vi "Turn Silver.vi"(8 "error in (no error)":errorcluster) -> (0 "error out":errorcluster)   [LabVIEW 2021]
uses:
  <vilib>/Utility/miscctls.llb/LVFontTypeDef.ctl
  <vilib>/Utility/miscctls.llb/LVPositionTypeDef.ctl
panel:
  out "Control Types on VI":string[](array[string])
  in  "vi path":path
  # "This VI will attempt to replace the front panel controls with their silver versions.  Not all controls are supported but you can follow the same steps to add support for other controls.\nNote that all DAQmx controls will be changed to Channel terminals, rather than Device terminals.\n\nThis VI is shamelessly stolen and edited from Hooovahh's great post here:\nhttps://forums.ni.com/t5/LabVIEW/Replace-cluster-bug/m-p/3148093/highlight/true#M906580"
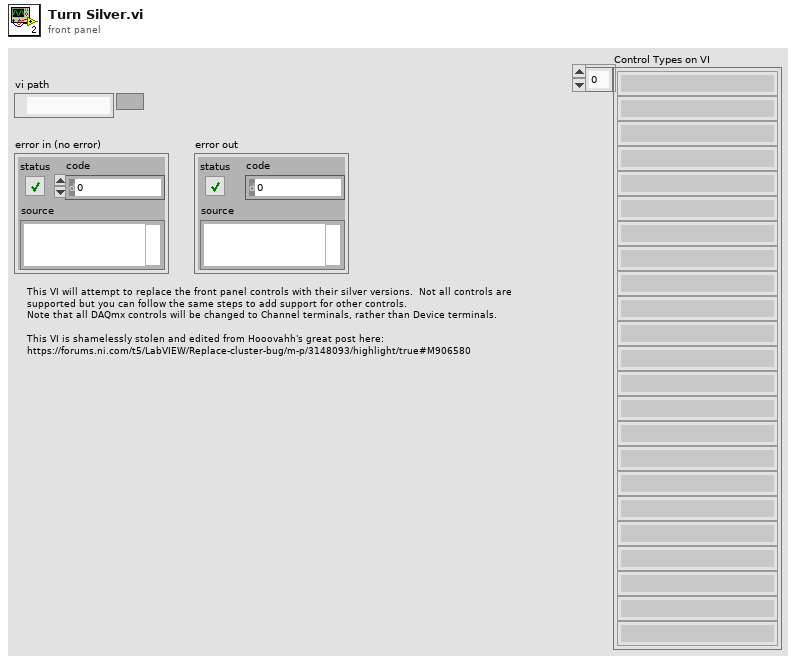
[diagram p1: front panel]
types:
  T1 = enum32{"Invalid", "Standard", "Closed", "Hidden", "Minimized", "Maximized"}
  T2 = typedef "LVFontTypeDef.ctl" = cluster{"Font Name":string, "Size":u16, "Bold":bool, "Italic":bool, "Underline":bool, "Strikeout":bool, "Color":u32}
  T3 = typedef "LVPositionTypeDef.ctl" = cluster{"Left":i32, "Top":i32}
  T4 = enum32{"not a typedef", "typedef", "strict typedef", "class private data"}
  T5 = typedef "LVBrowseOptionsTypeDef.ctl" = cluster{"Prompt":string, "Match Pattern":string, "select mode":enum32{"existing file", "new file", "new or existing file", "existing dir", "new dir", "new or existing dir", "existing file (use LLBs)", "new file (use LLBs)", "new or existing file (use LLBs)", "new or existing file or directory (use LLBs)", "existing dir (use LLBs)", "new dir (use LLBs)", "new or existing dir (use LLBs)", "existing file or dir", "new file or dir", "new or existing file or dir", "existing file or dir (use LLBs)", "new file or dir (use LLBs)"}, "Start Path":path, "Pattern Label":string, "Button Text":string}
  T6 = cluster{"left":i16, "top":i16, "right":i16, "bottom":i16}
  T7 = typedef "LVStringsAndValuesArrayTypeDef.ctl" = cluster{"String":string, "Value":ext}[]
  T8 = typedef "LVBoundsTypeDef.ctl" = cluster{"Width":u32, "Height":u32}
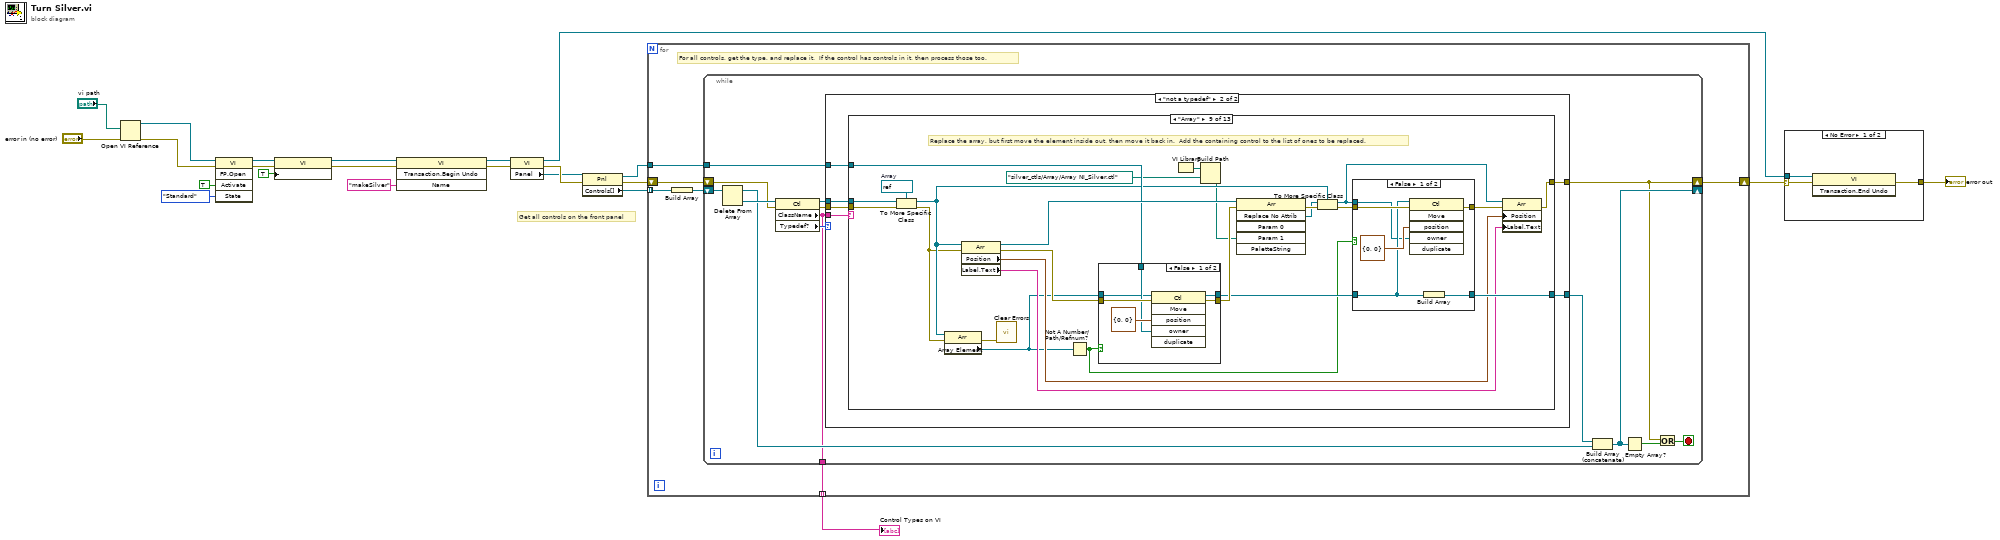
[diagram p0: block diagram]
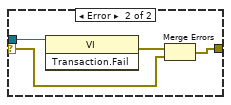
[diagram p2: hidden frame]
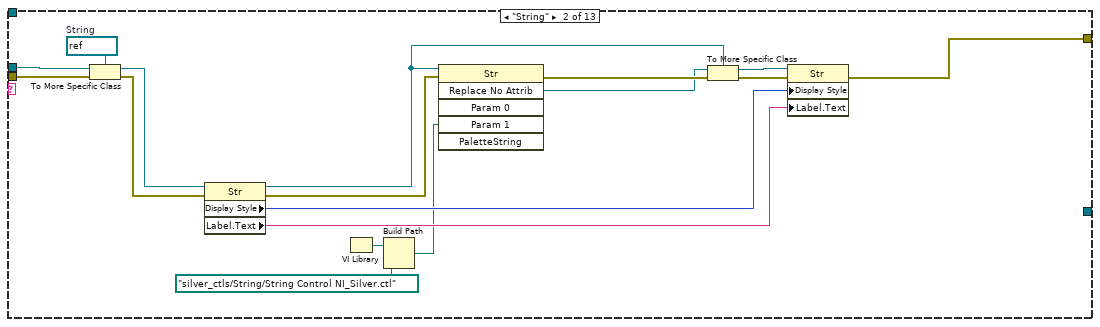
[diagram p5: hidden frame]
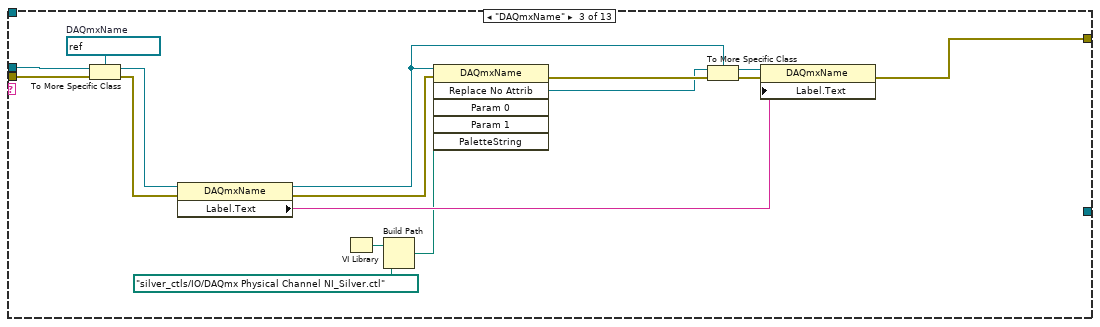
[diagram p6: hidden frame]
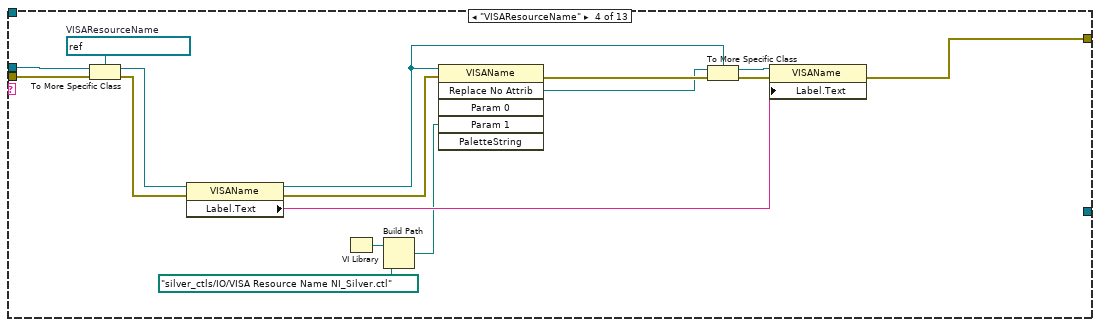
[diagram p7: hidden frame]
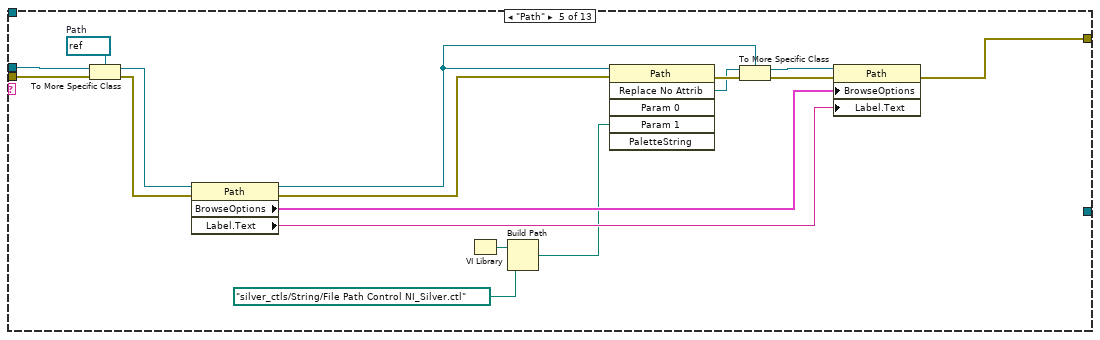
[diagram p8: hidden frame]
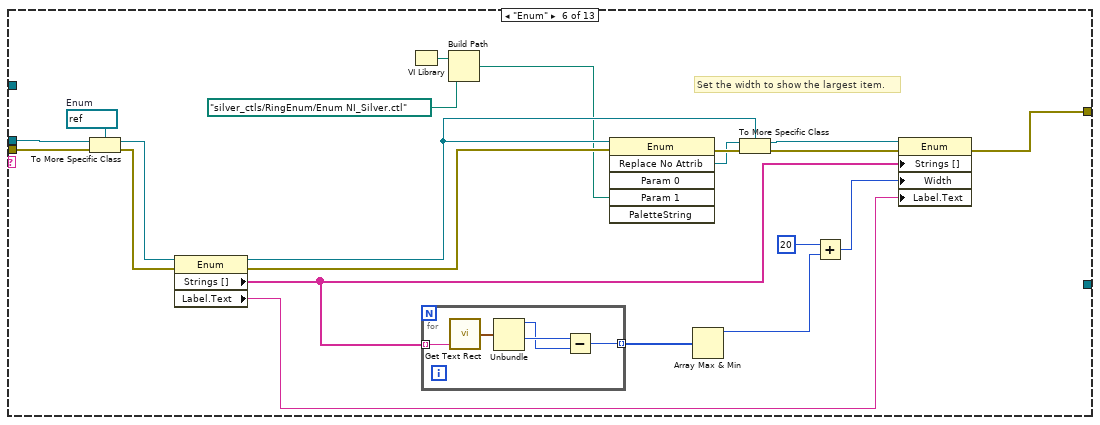
[diagram p9: hidden frame]
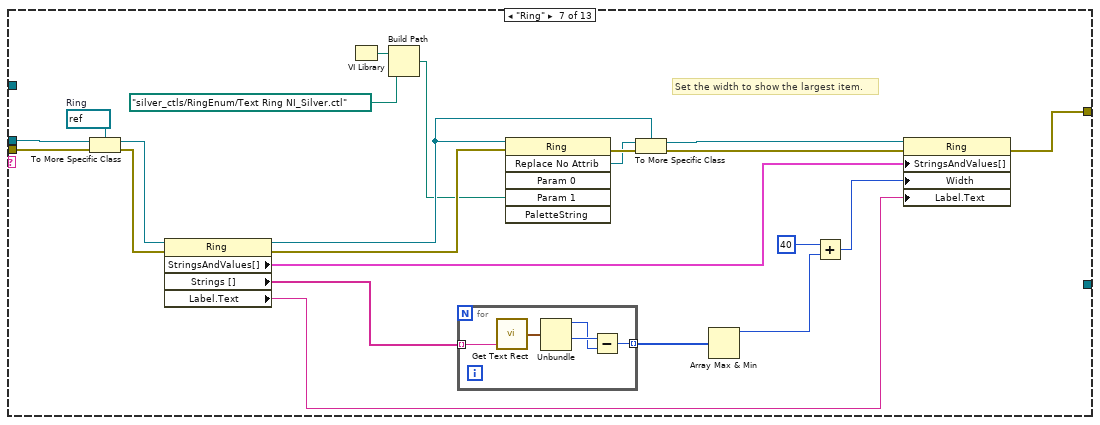
[diagram p10: hidden frame]
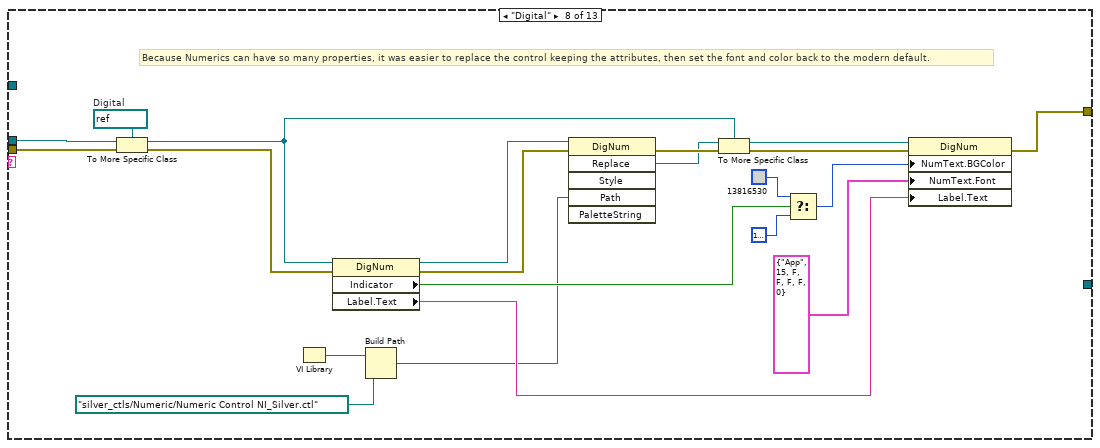
[diagram p11: hidden frame]
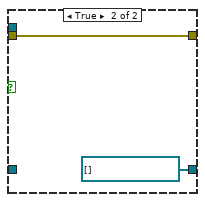
[diagram p12: hidden frame]
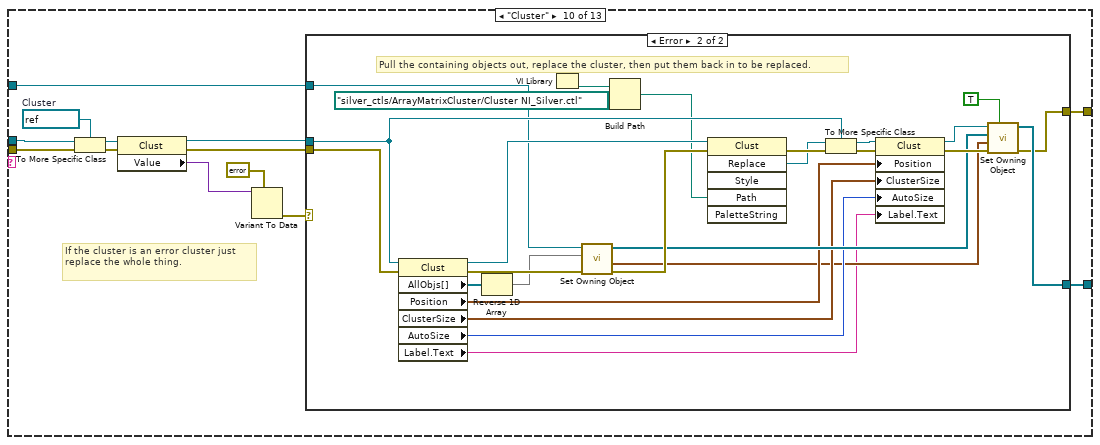
[diagram p14: hidden frame]
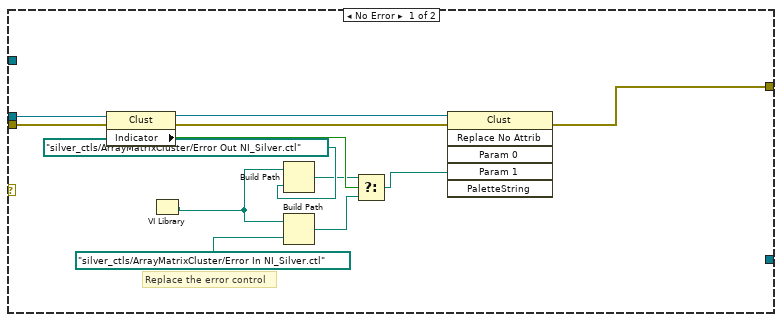
[diagram p15: hidden frame]
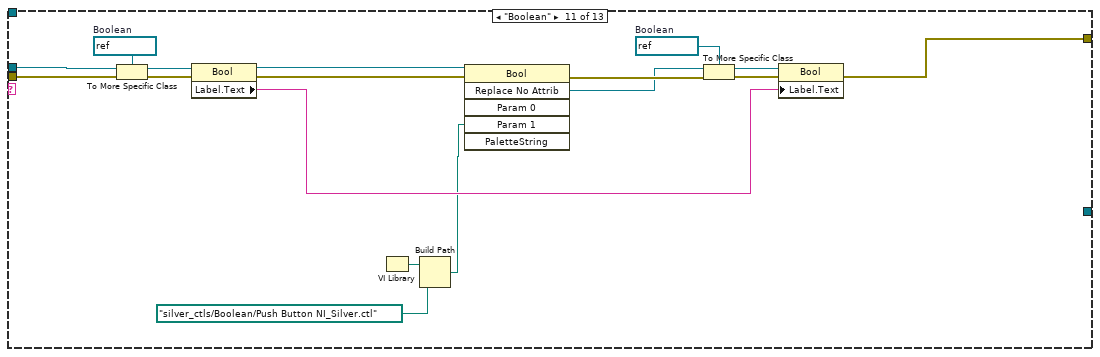
[diagram p16: hidden frame]
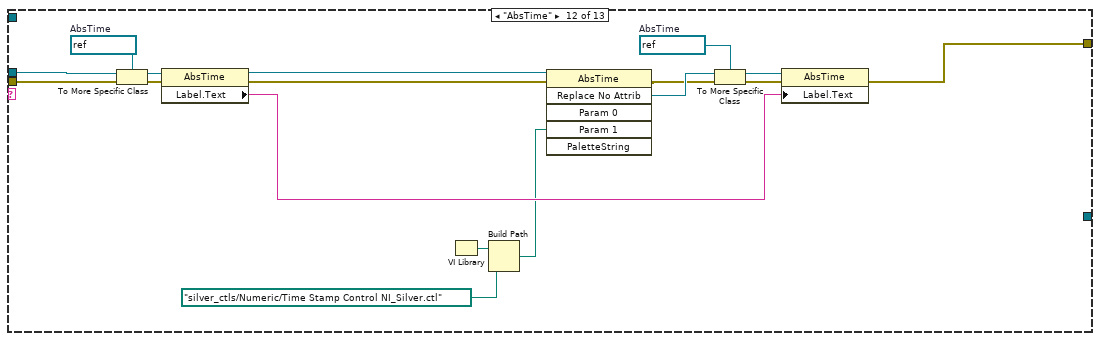
[diagram p17: hidden frame]
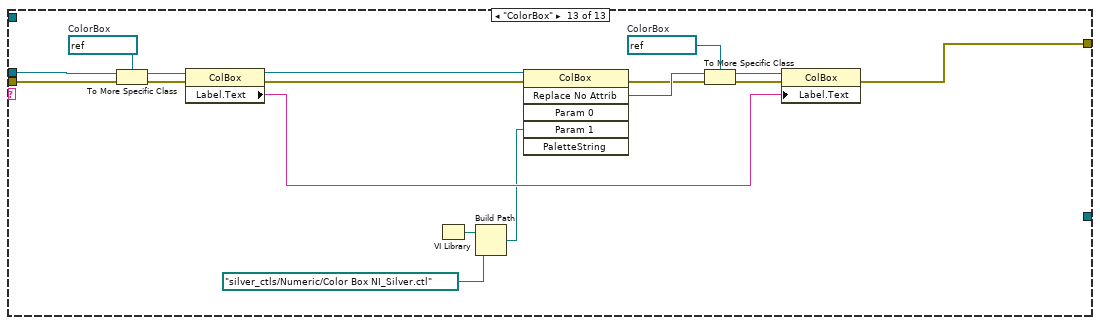
[diagram p18: hidden frame]
diagram:
  # "Get all controls on the front panel"
  n1 = Open VI Reference(vi path="vi path", error in (no error)="error in (no error)") -> (vi reference=w5:refnum<vi>, error out=w3:errorcluster)  [unwired: 4 in]
  n2 = invoke class="VI" method="FP.Open"(reference=w5, error in=w3, "Activate"=TRUE ("Activate?"), "State"=T1."Standard") -> (reference out=w11:refnum<vi>, error out=w12:errorcluster)  [unwired: 1 in, 3 out]
  n3 = property class="VI"(reference=w11, error in=w12, "Front Panel.IsFrontmost"=TRUE ("Front Panel Window:Is Frontmost")) -> (reference out=w6:refnum<vi>, error out=w7:errorcluster)
  n4 = invoke class="VI" method="Transaction.Begin Undo"(reference=w6, error in=w7, "Name"="makeSilver") -> (reference out=w17:refnum<vi>, error out=w18:errorcluster)  [unwired: 1 in, 2 out]
  n5 = property class="VI"(reference=w17, error in=w18) -> (reference out=w14:refnum<vi>, error out=w21:errorcluster, "Panel"=w20:refnum<vi>)
  n6 = property class="Pnl"(reference=w20, error in=w21) -> (reference out=w19:refnum<vi>, error out=w22:errorcluster, "Controls[]"=w23:refnum<vi>[])
  n7 = for {
    tunnel: w23 -> [w28] mode=indexing
    tunnel: w19 -> [w29]
    shift-right: [w25] -> w13
    shift-left: w22 -> [w26]
    tunnel: [w24] -> w1 mode=indexing
    # "For all controls, get the type, and replace it.  If the control has controls in it, then process those too."
    n8 = Build Array(w28) -> (w27:refnum<vi>[])
    n9 = while {
      tunnel: w29 -> [w43]
      shift-right: [w34] -> _
      shift-left: w27 -> [w38]
      shift-right: [w31] -> w25
      shift-left: w26 -> [w33]
      tunnel: [w30] -> w24
      stop <- w32 stop-if-true
      n10 = Delete From Array(array=w38) -> (deleted portion=w37:refnum<vi>, array with subset deleted=w35:refnum<vi>[])  [unwired: 2 in]
      n11 = property class="Ctl"(reference=w37, error in=w33) -> (reference out=w42:refnum<vi>, error out=w41:errorcluster, "ClassName"=w30:string, "Typedef?"=w40:T4)
      n12 = case shown="\"not a typedef\"" w40 {
        tunnel: w43 -> [_ w50]
        tunnel: w42 -> [_ w49]
        tunnel: w30 -> [_ w48]
        tunnel: w41 -> [w44 w47]
        tunnel: [_ w46] -> w36
        tunnel: [w44 w45] -> w31
        frame Default {
          # "Don't try to replace type defs."
        }
        frame "not a typedef" {
          n13 = case shown="\"Array\"" w48 {
            tunnel: w50 -> [_ _ _ _ _ _ _ _ w207 w241 _ _ _]
            tunnel: w49 -> [_ w68 w84 w100 w117 w138 w165 w191 w216 w245 w300 w317 w334]
            tunnel: w47 -> [w51 w62 w78 w94 w111 w134 w161 w187 w212 w243 w297 w314 w331]
            tunnel: [_ _ _ _ _ _ _ _ w205 w240 _ _ _] -> w46
            tunnel: [w51 w55 w72 w88 w104 w121 w147 w175 w201 w233 w288 w304 w321] -> w45
            frame Default {
            }
            frame "String" {
              w67 = refnum<vi> refnum  # String
              n14 = To More Specific Class(target class=w67, reference=w68, error in=w62) -> (specific class reference=w58:refnum<vi>, error out=w60:errorcluster)
              n15 = property class="Str"(reference=w58, error in=w60) -> (reference out=w57:refnum<vi>, error out=w59:errorcluster, "Display Style"=w61:u32, "Label.Text"=w56:string)
              n16 = VI Library() -> (path=w53:path)
              n17 = Build Path(base path=w53, name or relative path=path "silver_ctls/String/String Control NI_Silver.ctl" ("path")) -> (appended path=w52:path)
              n18 = invoke class="Str" method="Replace No Attrib"(reference=w57, error in=w59, "Param 1"=w52) -> (error out=w66:errorcluster, "RepNoAttrib"=w64:refnum<vi>)  [unwired: 3 in, 4 out]
              n19 = To More Specific Class(target class=w57, reference=w64, error in=w66) -> (specific class reference=w63:refnum<vi>, error out=w65:errorcluster)
              n20 = property class="Str"(reference=w63, error in=w65, "Display Style"=w61, "Label.Text"=w56) -> (error out=w55:errorcluster)  [unwired: 1 out]
            }
            frame "DAQmxName" {
              w83 = refnum<vi> refnum  # DAQmxName
              n21 = To More Specific Class(target class=w83, reference=w84, error in=w78) -> (specific class reference=w75:refnum<vi>, error out=w77:errorcluster)
              n22 = property class="DAQmxName"(reference=w75, error in=w77) -> (reference out=w74:refnum<vi>, error out=w76:errorcluster, "Label.Text"=w73:string)
              n23 = VI Library() -> (path=w70:path)
              n24 = Build Path(base path=w70, name or relative path=path "silver_ctls/IO/DAQmx Physical Channel NI_Silver.ctl" ("path")) -> (appended path=w69:path)
              n25 = invoke class="DAQmxName" method="Replace No Attrib"(reference=w74, error in=w76, "Param 1"=w69) -> (error out=w82:errorcluster, "RepNoAttrib"=w80:refnum<vi>)  [unwired: 3 in, 4 out]
              n26 = To More Specific Class(target class=w74, reference=w80, error in=w82) -> (specific class reference=w79:refnum<vi>, error out=w81:errorcluster)
              n27 = property class="DAQmxName"(reference=w79, error in=w81, "Label.Text"=w73) -> (error out=w72:errorcluster)  [unwired: 1 out]
            }
            frame "VISAResourceName" {
              w99 = refnum<vi> refnum  # VISAResourceName
              n28 = To More Specific Class(target class=w99, reference=w100, error in=w94) -> (specific class reference=w91:refnum<vi>, error out=w93:errorcluster)
              n29 = property class="VISAName"(reference=w91, error in=w93) -> (reference out=w90:refnum<vi>, error out=w92:errorcluster, "Label.Text"=w89:string)
              n30 = VI Library() -> (path=w86:path)
              n31 = Build Path(base path=w86, name or relative path=path "silver_ctls/IO/VISA Resource Name NI_Silver.ctl" ("path")) -> (appended path=w85:path)
              n32 = invoke class="VISAName" method="Replace No Attrib"(reference=w90, error in=w92, "Param 1"=w85) -> (error out=w98:errorcluster, "RepNoAttrib"=w96:refnum<vi>)  [unwired: 3 in, 4 out]
              n33 = To More Specific Class(target class=w90, reference=w96, error in=w98) -> (specific class reference=w95:refnum<vi>, error out=w97:errorcluster)
              n34 = property class="VISAName"(reference=w95, error in=w97, "Label.Text"=w89) -> (error out=w88:errorcluster)  [unwired: 1 out]
            }
            frame "Path" {
              w116 = refnum<vi> refnum  # Path
              n35 = To More Specific Class(target class=w116, reference=w117, error in=w111) -> (specific class reference=w107:refnum<vi>, error out=w109:errorcluster)
              n36 = property class="Path"(reference=w107, error in=w109) -> (reference out=w106:refnum<vi>, error out=w108:errorcluster, "BrowseOptions"=w110:T5, "Label.Text"=w105:string)
              n37 = VI Library() -> (path=w102:path)
              n38 = Build Path(base path=w102, name or relative path=path "silver_ctls/String/File Path Control NI_Silver.ctl" ("path")) -> (appended path=w101:path)
              n39 = invoke class="Path" method="Replace No Attrib"(reference=w106, error in=w108, "Param 1"=w101) -> (error out=w115:errorcluster, "RepNoAttrib"=w113:refnum<vi>)  [unwired: 3 in, 4 out]
              n40 = To More Specific Class(target class=w106, reference=w113, error in=w115) -> (specific class reference=w112:refnum<vi>, error out=w114:errorcluster)
              n41 = property class="Path"(reference=w112, error in=w114, "BrowseOptions"=w110, "Label.Text"=w105) -> (error out=w104:errorcluster)  [unwired: 1 out]
            }
            frame "Enum" {
              w137 = refnum<vi> refnum  # Enum
              # "Set the width to show the largest item."
              n42 = To More Specific Class(target class=w137, reference=w138, error in=w134) -> (specific class reference=w131:refnum<vi>, error out=w133:errorcluster)
              n43 = property class="Enum"(reference=w131, error in=w133) -> (reference out=w130:refnum<vi>, error out=w132:errorcluster, "Strings []"=w127:string[], "Label.Text"=w122:string)
              n44 = VI Library() -> (path=w119:path)
              n45 = for {
                tunnel: w127 -> [w143] mode=indexing
                tunnel: [w139] -> w126 mode=indexing
                n46 = call <vilib>:"Get Text Rect.vi"("text"=w143) -> ("rect"=w140:T6)  [unwired: 8 in]
                n47 = Unbundle(w140) -> ("left"=w141:i16, "right"=w142:i16)  [unwired: 2 out]
                n48 = Subtract(x=w142, y=w141) -> (x-y=w139:i16)
              }
              n49 = Build Path(base path=w119, name or relative path=path "silver_ctls/RingEnum/Enum NI_Silver.ctl" ("path")) -> (appended path=w118:path)
              n50 = invoke class="Enum" method="Replace No Attrib"(reference=w130, error in=w132, "Param 1"=w118) -> (error out=w136:errorcluster, "RepNoAttrib"=w135:refnum<vi>)  [unwired: 3 in, 4 out]
              n51 = Array Max & Min(array=w126) -> (max value=w125:i16)  [unwired: 3 out]
              n52 = To More Specific Class(target class=w130, reference=w135, error in=w136) -> (specific class reference=w129:refnum<vi>, error out=w128:errorcluster)
              n53 = Add(x=i16 20, y=w125) -> (x+y=w124:i16)
              n54 = property class="Enum"(reference=w129, error in=w128, "Strings []"=w127, "Width"=w124, "Label.Text"=w122) -> (error out=w121:errorcluster)  [unwired: 1 out]
            }
            frame "Ring" {
              w164 = refnum<vi> refnum  # Ring
              # "Set the width to show the largest item."
              n55 = To More Specific Class(target class=w164, reference=w165, error in=w161) -> (specific class reference=w158:refnum<vi>, error out=w160:errorcluster)
              n56 = property class="Ring"(reference=w158, error in=w160) -> (reference out=w157:refnum<vi>, error out=w159:errorcluster, "StringsAndValues[]"=w149:T7, "Strings []"=w150:string[], "Label.Text"=w148:string)
              n57 = VI Library() -> (path=w145:path)
              n58 = Build Path(base path=w145, name or relative path=path "silver_ctls/RingEnum/Text Ring NI_Silver.ctl" ("path")) -> (appended path=w144:path)
              n59 = for {
                tunnel: w150 -> [w170] mode=indexing
                tunnel: [w166] -> w154 mode=indexing
                n60 = call <vilib>:"Get Text Rect.vi"("text"=w170) -> ("rect"=w167:T6)  [unwired: 8 in]
                n61 = Unbundle(w167) -> ("left"=w168:i16, "right"=w169:i16)  [unwired: 2 out]
                n62 = Subtract(x=w169, y=w168) -> (x-y=w166:i16)
              }
              n63 = invoke class="Ring" method="Replace No Attrib"(reference=w157, error in=w159, "Param 1"=w144) -> (error out=w163:errorcluster, "RepNoAttrib"=w162:refnum<vi>)  [unwired: 3 in, 4 out]
              n64 = To More Specific Class(target class=w157, reference=w162, error in=w163) -> (specific class reference=w156:refnum<vi>, error out=w155:errorcluster)
              n65 = Array Max & Min(array=w154) -> (max value=w153:i16)  [unwired: 3 out]
              n66 = Add(x=i16 40, y=w153) -> (x+y=w152:i16)
              n67 = property class="Ring"(reference=w156, error in=w155, "StringsAndValues[]"=w149, "Width"=w152, "Label.Text"=w148) -> (error out=w147:errorcluster)  [unwired: 1 out]
            }
            frame "Digital" {
              w190 = refnum<vi> refnum  # Digital
              # "Because Numerics can have so many properties, it was easier to replace the control keeping the attributes, then set the font and color back to the modern default."
              n68 = To More Specific Class(target class=w190, reference=w191, error in=w187) -> (specific class reference=w179:refnum<vi>, error out=w177:errorcluster)
              n69 = VI Library() -> (path=w172:path)
              n70 = property class="DigNum"(reference=w179, error in=w177) -> (reference out=w178:refnum<vi>, error out=w176:errorcluster, "Indicator"=w183:bool, "Label.Text"=w174:string)
              n71 = Build Path(base path=w172, name or relative path=path "silver_ctls/Numeric/Numeric Control NI_Silver.ctl" ("path")) -> (appended path=w171:path)
              n72 = invoke class="DigNum" method="Replace"(reference=w178, error in=w176, "Path"=w171) -> (error out=w189:errorcluster, "Replace"=w188:refnum<vi>)  [unwired: 3 in, 4 out]
              n73 = To More Specific Class(target class=w179, reference=w188, error in=w189) -> (specific class reference=w185:refnum<vi>, error out=w186:errorcluster)
              n74 = Select(t=u32 13816530, s=w183, f=u32 16777226) -> (s? t:f=w180:u32)
              n75 = property class="DigNum"(reference=w185, error in=w186, "NumText.BGColor"=w180, "NumText.Font"=T2 {"Font Name"="App", "Size"=15, "Bold"=FALSE, "Italic"=FALSE, "Underline"=FALSE, "Strikeout"=FALSE, "Color"=0} ("Numeric Text.Font"), "Label.Text"=w174) -> (error out=w175:errorcluster)  [unwired: 1 out]
            }
            frame "Array" {
              w215 = refnum<vi> refnum  # Array
              # "Replace the array, but first move the element inside out, then move it back in.  Add the containing control to the list of ones to be replaced."
              n76 = To More Specific Class(target class=w215, reference=w216, error in=w212) -> (specific class reference=w200:refnum<vi>, error out=w199:errorcluster)
              n77 = property class="Arr"(reference=w200, error in=w199) -> (error out=w195:errorcluster, "Array Element"=w198:refnum<vi>)  [unwired: 1 out]
              n78 = property class="Arr"(reference=w200, error in=w199) -> (reference out=w211:refnum<vi>, error out=w210:errorcluster, "Position"=w203:T3, "Label.Text"=w202:string)
              n79 = call <vilib>:"Clear Errors.vi"("error in (no error)"=w195) -> ()  [unwired: 5 in, 2 out]
              n80 = Not A Number/Path/Refnum?(number/path/refnum=w198) -> (NaN/Path/Refnum?=w196:bool)
              n81 = case shown="False" w196 {
                tunnel: w210 -> [w230 w232]
                tunnel: [w229 w232] -> w209
                tunnel: w207 -> [w227 _]
                tunnel: [w226 w231] -> w206
                tunnel: w198 -> [w225 w231]
                frame False {
                  n82 = invoke class="Ctl" method="Move"(reference=w225, error in=w230, "position"=T3 {"Left"=0, "Top"=0}, "owner"=w227) -> (reference out=w226:refnum<vi>, error out=w229:errorcluster)  [unwired: 2 in, 4 out]
                }
                frame True {
                }
              }
              n83 = VI Library() -> (path=w193:path)
              n84 = Build Path(base path=w193, name or relative path=path "silver_ctls/Array/Array NI_Silver.ctl" ("path")) -> (appended path=w192:path)
              n85 = invoke class="Arr" method="Replace No Attrib"(reference=w211, error in=w209, "Param 1"=w192) -> (error out=w214:errorcluster, "RepNoAttrib"=w213:refnum<vi>)  [unwired: 3 in, 4 out]
              n86 = To More Specific Class(target class=w200, reference=w213, error in=w214) -> (specific class reference=w197:refnum<vi>, error out=w208:errorcluster)
              n87 = case shown="False" w196 {
                tunnel: w208 -> [w221 w224]
                tunnel: w206 -> [w220 _]
                tunnel: [w219 refnum<vi>[] []] -> w205
                tunnel: w197 -> [w218 _]
                tunnel: [w217 w224] -> w204
                frame False {
                  n88 = invoke class="Ctl" method="Move"(reference=w220, error in=w221, "position"=T3 {"Left"=0, "Top"=0}, "owner"=w218) -> (error out=w217:errorcluster)  [unwired: 2 in, 5 out]
                  n89 = Build Array(w220) -> (w219:refnum<vi>[])
                }
                frame True {
                }
              }
              n90 = property class="Arr"(reference=w197, error in=w204, "Position"=w203, "Label.Text"=w202) -> (error out=w201:errorcluster)  [unwired: 1 out]
            }
            frame "Cluster" {
              w244 = refnum<vi> refnum  # Cluster
              # "If the cluster is an error cluster just replace the whole thing."
              n91 = To More Specific Class(target class=w244, reference=w245, error in=w243) -> (specific class reference=w238:refnum<vi>, error out=w242:errorcluster)
              n92 = property class="Clust"(reference=w238, error in=w242) -> (reference out=w237:refnum<vi>, error out=w239:errorcluster, "Value"=w236:variant)
              n93 = Variant To Data(type=errorcluster {"status"=FALSE, "code"=0, "source"=""} ("error in (no error)"), Variant=w236) -> (error out=w234:errorcluster)  [unwired: 1 in, 1 out]
              n94 = case shown="Error" w234 {
                tunnel: w237 -> [w255 w281]
                tunnel: w239 -> [w257 w279]
                tunnel: w241 -> [_ w276]
                tunnel: [_ w264] -> w240
                tunnel: [w247 w262] -> w233
                frame No Error {
                  # "Replace the error control"
                  n95 = property class="Clust"(reference=w255, error in=w257) -> (reference out=w254:refnum<vi>, error out=w256:errorcluster, "Indicator"=w251:bool)
                  n96 = VI Library() -> (path=w246:path)
                  n97 = Build Path(base path=w246, name or relative path=path "silver_ctls/ArrayMatrixCluster/Error Out NI_Silver.ctl") -> (appended path=w250:path)
                  n98 = Build Path(base path=w246, name or relative path=path "silver_ctls/ArrayMatrixCluster/Error In NI_Silver.ctl") -> (appended path=w249:path)
                  n99 = Select(t=w250, s=w251, f=w249) -> (s? t:f=w248:path)
                  n100 = invoke class="Clust" method="Replace No Attrib"(reference=w254, error in=w256, "Param 1"=w248) -> (error out=w247:errorcluster)  [unwired: 3 in, 5 out]
                }
                frame Error {
                  # "Pull the containing objects out, replace the cluster, then put them back in to be replaced."
                  n101 = property class="Clust"(reference=w281, error in=w279) -> (reference out=w280:refnum<vi>, error out=w278:errorcluster, "AllObjs[]"=w266:refnum<vi>[], "Position"=w269:T3, "ClusterSize"=w270:T8, "AutoSize"=w271:u32, "Label.Text"=w261:string)
                  n102 = Reverse 1D Array(array=w266) -> (reversed array=w263:refnum<vi>[])
                  n103 = VI Library() -> (path=w259:path)
                  n104 = call "Set Owning Object.vi"("error in (no error)"=w278, "All Controls In"=w263, "Owner Object"=w276) -> ("error out"=w277:errorcluster, "Positions"=w268:T3[], "All Controls Out"=w272:refnum<vi>[])  [unwired: 6 in]
                  n105 = Build Path(base path=w259, name or relative path=path "silver_ctls/ArrayMatrixCluster/Cluster NI_Silver.ctl") -> (appended path=w258:path)
                  n106 = invoke class="Clust" method="Replace"(reference=w280, error in=w277, "Path"=w258) -> (error out=w283:errorcluster, "Replace"=w282:refnum<vi>)  [unwired: 3 in, 4 out]
                  n107 = To More Specific Class(target class=w281, reference=w282, error in=w283) -> (specific class reference=w275:refnum<vi>, error out=w274:errorcluster)
                  n108 = property class="Clust"(reference=w275, error in=w274, "Position"=w269, "ClusterSize"=w270, "AutoSize"=w271, "Label.Text"=w261) -> (reference out=w265:refnum<vi>, error out=w273:errorcluster)
                  n109 = call "Set Owning Object.vi"("Set Absolute"=TRUE, "error in (no error)"=w273, "Absolute Positions"=w268, "All Controls In"=w272, "Owner Object"=w265) -> ("error out"=w262:errorcluster, "All Controls Out"=w264:refnum<vi>[])  [unwired: 4 in, 1 out]
                }
              }
            }
            frame "Boolean" {
              w291 = refnum<vi> refnum  # Boolean
              w299 = refnum<vi> refnum  # Boolean
              n110 = To More Specific Class(target class=w299, reference=w300, error in=w297) -> (specific class reference=w295:refnum<vi>, error out=w298:errorcluster)
              n111 = property class="Bool"(reference=w295, error in=w298) -> (reference out=w294:refnum<vi>, error out=w296:errorcluster, "Label.Text"=w287:string)
              n112 = VI Library() -> (path=w285:path)
              n113 = Build Path(base path=w285, name or relative path=path "silver_ctls/Boolean/Push Button NI_Silver.ctl" ("path")) -> (appended path=w284:path)
              n114 = invoke class="Bool" method="Replace No Attrib"(reference=w294, error in=w296, "Param 1"=w284) -> (error out=w290:errorcluster, "RepNoAttrib"=w289:refnum<vi>)  [unwired: 3 in, 4 out]
              n115 = To More Specific Class(target class=w291, reference=w289, error in=w290) -> (specific class reference=w293:refnum<vi>, error out=w292:errorcluster)
              n116 = property class="Bool"(reference=w293, error in=w292, "Label.Text"=w287) -> (error out=w288:errorcluster)  [unwired: 1 out]
            }
            frame "AbsTime" {
              w308 = refnum<vi> refnum  # AbsTime
              w316 = refnum<vi> refnum  # AbsTime
              n117 = To More Specific Class(target class=w316, reference=w317, error in=w314) -> (specific class reference=w312:refnum<vi>, error out=w315:errorcluster)
              n118 = property class="AbsTime"(reference=w312, error in=w315) -> (reference out=w311:refnum<vi>, error out=w313:errorcluster, "Label.Text"=w305:string)
              n119 = VI Library() -> (path=w302:path)
              n120 = Build Path(base path=w302, name or relative path=path "silver_ctls/Numeric/Time Stamp Control NI_Silver.ctl" ("path")) -> (appended path=w301:path)
              n121 = invoke class="AbsTime" method="Replace No Attrib"(reference=w311, error in=w313, "Param 1"=w301) -> (error out=w306:errorcluster, "RepNoAttrib"=w307:refnum<vi>)  [unwired: 3 in, 4 out]
              n122 = To More Specific Class(target class=w308, reference=w307, error in=w306) -> (specific class reference=w310:refnum<vi>, error out=w309:errorcluster)
              n123 = property class="AbsTime"(reference=w310, error in=w309, "Label.Text"=w305) -> (error out=w304:errorcluster)  [unwired: 1 out]
            }
            frame "ColorBox" {
              w325 = refnum<vi> refnum  # ColorBox
              w333 = refnum<vi> refnum  # ColorBox
              n124 = To More Specific Class(target class=w333, reference=w334, error in=w331) -> (specific class reference=w329:refnum<vi>, error out=w332:errorcluster)
              n125 = property class="ColBox"(reference=w329, error in=w332) -> (reference out=w328:refnum<vi>, error out=w330:errorcluster, "Label.Text"=w322:string)
              n126 = VI Library() -> (path=w319:path)
              n127 = Build Path(base path=w319, name or relative path=path "silver_ctls/Numeric/Color Box NI_Silver.ctl" ("path")) -> (appended path=w318:path)
              n128 = invoke class="ColBox" method="Replace No Attrib"(reference=w328, error in=w330, "Param 1"=w318) -> (error out=w323:errorcluster, "RepNoAttrib"=w324:refnum<vi>)  [unwired: 3 in, 4 out]
              n129 = To More Specific Class(target class=w325, reference=w324, error in=w323) -> (specific class reference=w327:refnum<vi>, error out=w326:errorcluster)
              n130 = property class="ColBox"(reference=w327, error in=w326, "Label.Text"=w322) -> (error out=w321:errorcluster)  [unwired: 1 out]
            }
          }
        }
      }
      n131 = Build Array (concatenate)(w36, w35) -> (w34:refnum<vi>[])
      n132 = Empty Array?(array=w34) -> (empty?=w39:bool)
      n133 = Or(x=w31, y=w39) -> (x .or. y?=w32:bool)
    }
  }
  "Control Types on VI" <- w1
  n134 = case shown="No Error" w13 {
    selector: w13 -> [w337 w338]
    tunnel: [w335 w339] -> w15
    tunnel: w14 -> [w336 w340]
    frame No Error {
      n135 = invoke class="VI" method="Transaction.End Undo"(reference=w336, error in=w337) -> (error out=w335:errorcluster)  [unwired: 1 in, 2 out]
    }
    frame Error {
      n136 = invoke class="VI" method="Transaction.Fail"(reference=w340) -> (error out=w341:errorcluster)  [unwired: 2 in, 2 out]
      n137 = Merge Errors(w341, w338) -> (w339:errorcluster)
    }
  }
  "error out" <- w15
